vi "WC_Drive_Fill Motion Buffers.vi"(7 "MotionProfiles":T6, 8 "Error":errorcluster, 10 "Buffer Status Array":T8[](array[typedef]), 11 "RobotDriveDevRef":T1) -> (0 "Error Out":errorcluster, 2 "Buffer Status Array Out":T8[](array[typedef]), 3 "RobotDriveDevRef Out":T1, 5 "Buffers Full Out":bool)   [LabVIEW 2016, in "WC_Drive.lvlib"]
uses:
  WC_Drive.lvlib
  TypeDef/ENUM_Drive_SRX Motion Buffer Status.ctl
  TypeDef/CLUSTER_Drive_Motion Profile Arrays.ctl
  TypeDef/CLUSTER_Drive_Point Specification.ctl
  <vilib>/Rock Robotics/WPI/RobotDrive/WPI_RobotDriveDevRef.ctl
  <vilib>/Rock Robotics/WPI/MotorControl/WPI_MotorControlDeviceRef.ctl
  <vilib>/Rock Robotics/WPI/MotorControl/WPI_MotorControlType.ctl
  <vilib>/Rock Robotics/SystemInterfaces/DIO/FPGA_DIOPWMChannel.ctl
  <vilib>/Rock Robotics/WPI/PWM/WPI_PWMDeadband.ctl
  TypeDef/ENUM_Drive_Side Select.ctl
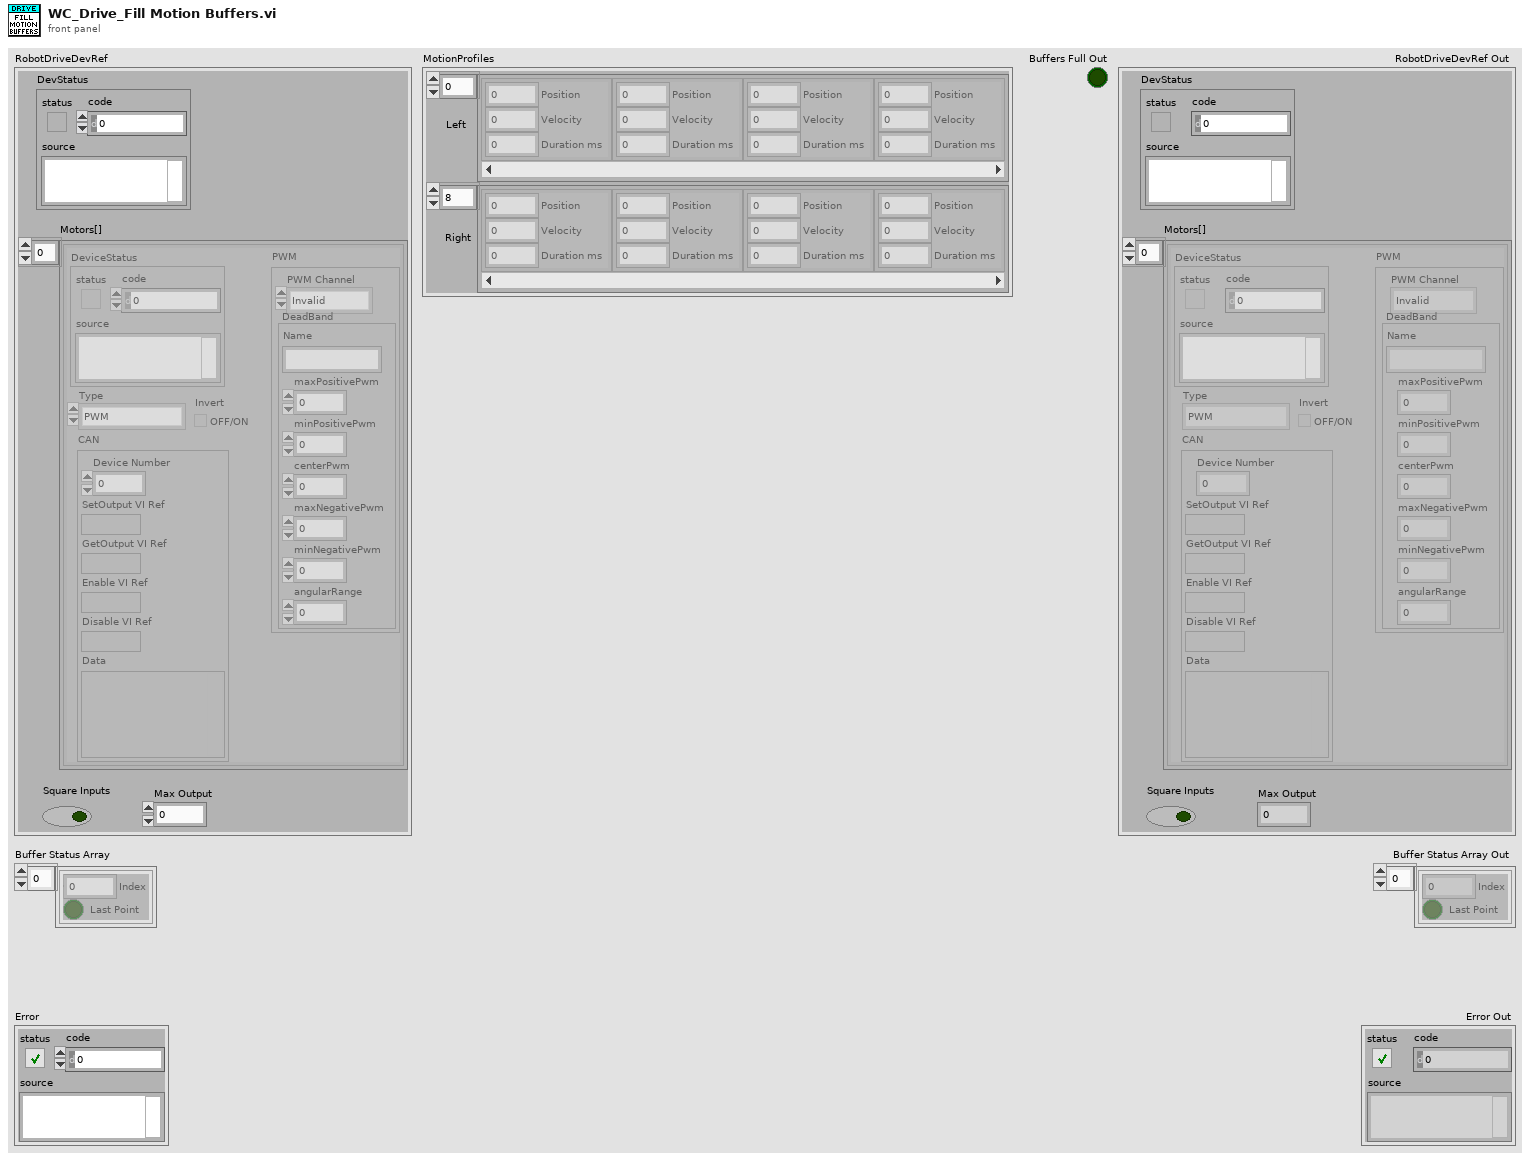
[diagram p1: front panel]
types:
  T1 = typedef "WPI_RobotDriveDevRef.ctl" = cluster{"DevStatus":errorcluster, "Motors[]":T2[], "Square Inputs":bool, "Max Output":dbl}
  T2 = typedef "WPI_MotorControlDeviceRef.ctl" = cluster{"DeviceStatus":errorcluster, "Type":T3, "PWM":cluster{"PWM Channel":T4, "DeadBand":T5}, "CAN":cluster{"Device Number":u8, "SetOutput VI Ref":variant, "GetOutput VI Ref":variant, "Enable VI Ref":variant, "Disable VI Ref":variant, "Data":variant}, "Invert":bool}
  T3 = typedef "WPI_MotorControlType.ctl" = enum16{"PWM", "CAN"}
  T4 = typedef "FPGA_DIOPWMChannel.ctl" = enum8{"PWM 0", "PWM 1", "PWM 2", "PWM 3", "PWM 4", "PWM 5", "PWM 6", "PWM 7", "PWM 8", "PWM 9", "PWM MXP 0", "PWM MXP 1", "PWM MXP 2", "PWM MXP 3", "PWM MXP 4", "PWM MXP 5", "PWM MXP 6", "PWM MXP 7", "PWM MXP 8", "PWM MXP 9", "Invalid"}
  T5 = typedef "WPI_PWMDeadband.ctl" = cluster{"Name":string, "maxPositivePwm":i32, "minPositivePwm":i32, "centerPwm":i32, "maxNegativePwm":i32, "minNegativePwm":i32, "angularRange":u16}
  T6 = typedef "CLUSTER_Drive_Motion Profile Arrays.ctl" = cluster{"Left":T7[], "Right":T7[]}
  T7 = typedef "CLUSTER_Drive_Point Specification.ctl" = cluster{"Position":dbl, "Velocity":dbl, "Duration ms":u8}
  T8 = typedef "ENUM_Drive_SRX Motion Buffer Status.ctl" = cluster{"Index":i32, "Last Point":bool}
  T9 = typedef "ENUM_Drive_Side Select.ctl" = enum16{"Left", "Right"}
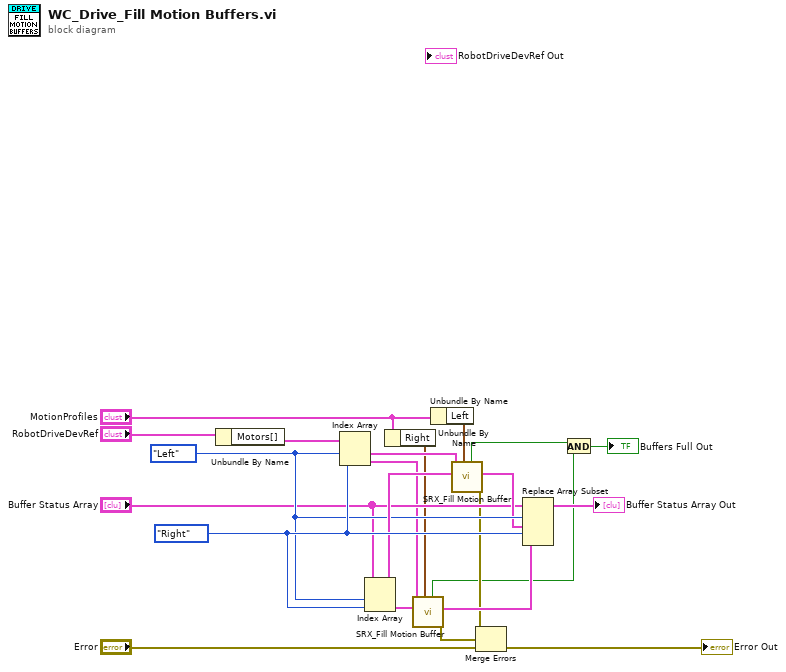
[diagram p0: block diagram]
diagram:
  w21 = ENUM_Drive_Side_Select."Right" ("Drive Side")
  w19 = ENUM_Drive_Side_Select."Left" ("Drive Side")
  n1 = Unbundle By Name("RobotDriveDevRef") -> ("Motors[]"=w9:T2[])
  n2 = Index Array(array=w9, index #1=w19, index #2=w21) -> (element #1=w13:T2, element #2=w14:T2)
  n3 = Index Array(array="Buffer Status Array", index #1=w19, index #2=w21) -> (element #1=w20:T8, element #2=w15:T8)
  n4 = Unbundle By Name("MotionProfiles") -> ("Right"=w12:T7[])
  n5 = call "SRX_Fill Motion Buffer.vi"("Profile Array"=w12, "Motion Buffer Status"=w15, "SingleMotorRef"=w14) -> ("Error Out"=w5:errorcluster, "Motion Buffer Status Out"=w18:T8, "Buffer Full Out"=w3:bool)  [unwired: 5 in, 1 out]
  n6 = Unbundle By Name("MotionProfiles") -> ("Left"=w11:T7[])
  n7 = call "SRX_Fill Motion Buffer.vi"("Profile Array"=w11, "Motion Buffer Status"=w20, "SingleMotorRef"=w13) -> ("Error Out"=w4:errorcluster, "Motion Buffer Status Out"=w17:T8, "Buffer Full Out"=w2:bool)  [unwired: 5 in, 1 out]
  n8 = Merge Errors(w4, w5, "Error") -> (→"Error Out":errorcluster)
  n9 = Replace Array Subset(array="Buffer Status Array", new element #1=w17, index #1=w19, new element #2=w18, index #2=w21) -> (→"Buffer Status Array Out":T8[])
  n10 = And(x=w2, y=w3) -> (x .and. y?=→"Buffers Full Out":bool)
